vi "OnMMove.vi"(0 "Start Goal Data":T1, 5 "x1 4":i32, 7 "x1 3":i32, 9 "x1 2":i32, 11 "x1":i32) -> (4 "Start Goal Data out":T1, 6 "x out":i32, 8 "y out":i32, 10 "Boolean":bool, 13 "x current -1":i32, 14 "y current -1":i32)   [LabVIEW 2013]
uses:
  Bug_StartGoalData.ctl
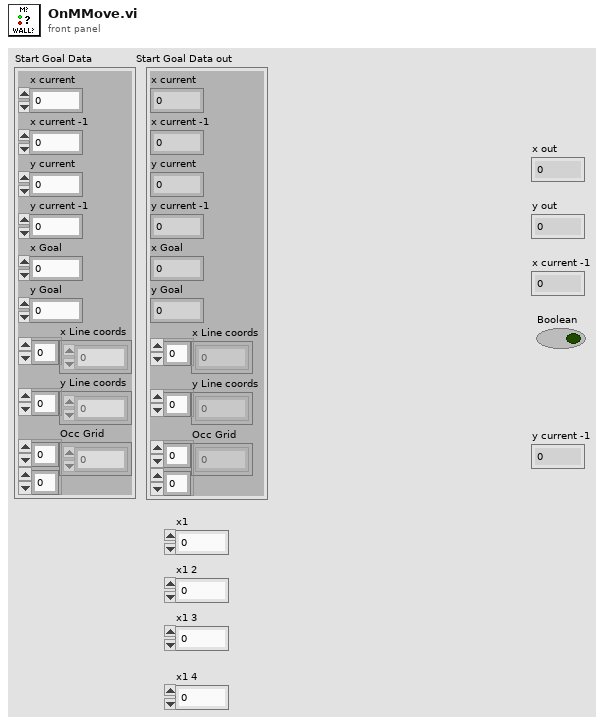
[diagram p1: front panel]
types:
  T1 = typedef "Bug_StartGoalData.ctl" = cluster{"x current":i32, "x current -1":i32, "y current":i32, "y current -1":i32, "x Goal":i32, "y Goal":i32, "x Line coords":i32[], "y Line coords":i32[], "Occ Grid":dbl[][]}
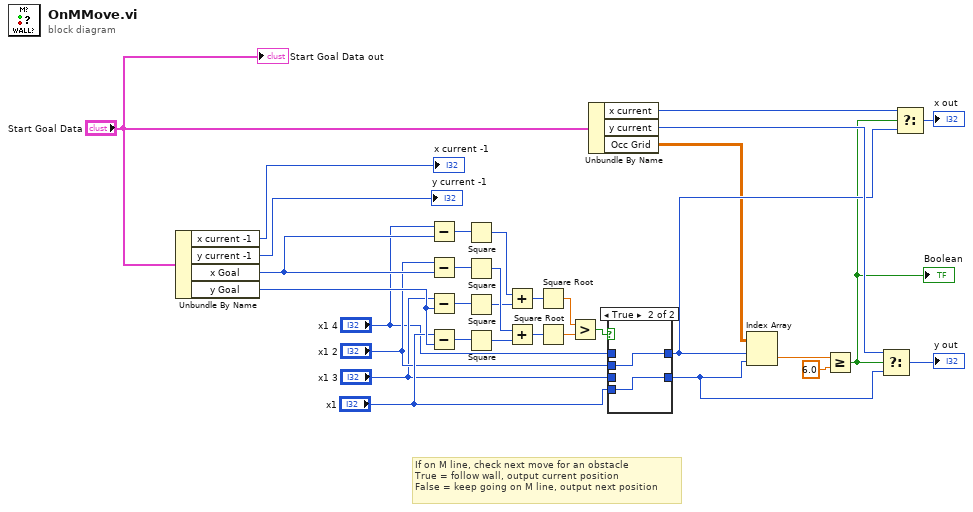
[diagram p0: block diagram]
diagram:
  # "If on M line, check next move for an obstacle\nTrue = follow wall, output current position\nFalse = keep going on M line, output next position"
  n1 = Unbundle By Name("Start Goal Data") -> ("x current -1"=→"x current -1":i32, "y current -1"=→"y current -1":i32, "x Goal"=w31:i32, "y Goal"=w32:i32)
  n2 = Subtract(x="x1 4", y=w31) -> (x-y=w8:i32)
  n3 = Subtract(x="x1 2", y=w31) -> (x-y=w10:i32)
  n4 = Subtract(x="x1 3", y=w32) -> (x-y=w9:i32)
  n5 = Subtract(x="x1", y=w32) -> (x-y=w11:i32)
  n6 = Square(x=w8) -> (x^2=w12:i32)
  n7 = Square(x=w10) -> (x^2=w14:i32)
  n8 = Square(x=w9) -> (x^2=w13:i32)
  n9 = Square(x=w11) -> (x^2=w15:i32)
  n10 = Add(x=w12, y=w13) -> (x+y=w16:i32)
  n11 = Add(x=w14, y=w15) -> (x+y=w17:i32)
  n12 = Square Root(x=w16) -> (sqrt(x)=w18:dbl)
  n13 = Square Root(x=w17) -> (sqrt(x)=w23:dbl)
  n14 = Greater?(x=w18, y=w23) -> (0:w19:bool)
  n15 = Unbundle By Name("Start Goal Data") -> ("x current"=w27:i32, "y current"=w28:i32, "Occ Grid"=w1:dbl[][])
  n16 = case shown="True" w19 {
    tunnel: "x1 4" -> [w34 _]
    tunnel: "x1 3" -> [w33 _]
    tunnel: "x1 2" -> [_ w36]
    tunnel: "x1" -> [_ w35]
    tunnel: [w34 w36] -> w25
    tunnel: [w33 w35] -> w26
    frame False {
    }
    frame True {
    }
  }
  n17 = Index Array(array=w1, index (row)=w25, index (col)=w26) -> (element=w3:dbl)
  n18 = Greater Or Equal?(x=w3, y=6.0) -> (x >= y?=w5:bool)
  "Boolean" <- w5
  n19 = Select(t=w28, s=w5, f=w26) -> (s? t:f=→"y out":i32)
  n20 = Select(t=w27, s=w5, f=w25) -> (s? t:f=→"x out":i32)
  "Start Goal Data out" <- "Start Goal Data"
